vi "Двоич-дес шф.vi"(0 "Registr":T3, 1 "Sign":bool) -> (2 "Segmen 2":T1, 3 "Segmen 1":T2)   [LabVIEW 2017]
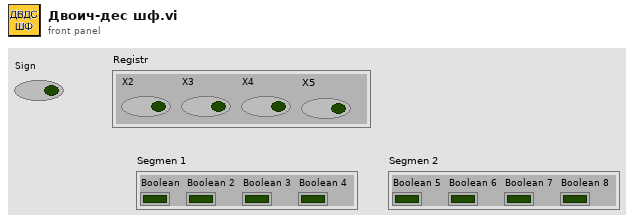
[diagram p1: front panel]
types:
  T1 = cluster{"Boolean 5":bool, "Boolean 6":bool, "Boolean 7":bool, "Boolean 8":bool}
  T2 = cluster{"Boolean":bool, "Boolean 2":bool, "Boolean 3":bool, "Boolean 4":bool}
  T3 = cluster{"X2":bool, "X3":bool, "X4":bool, "X5":bool}
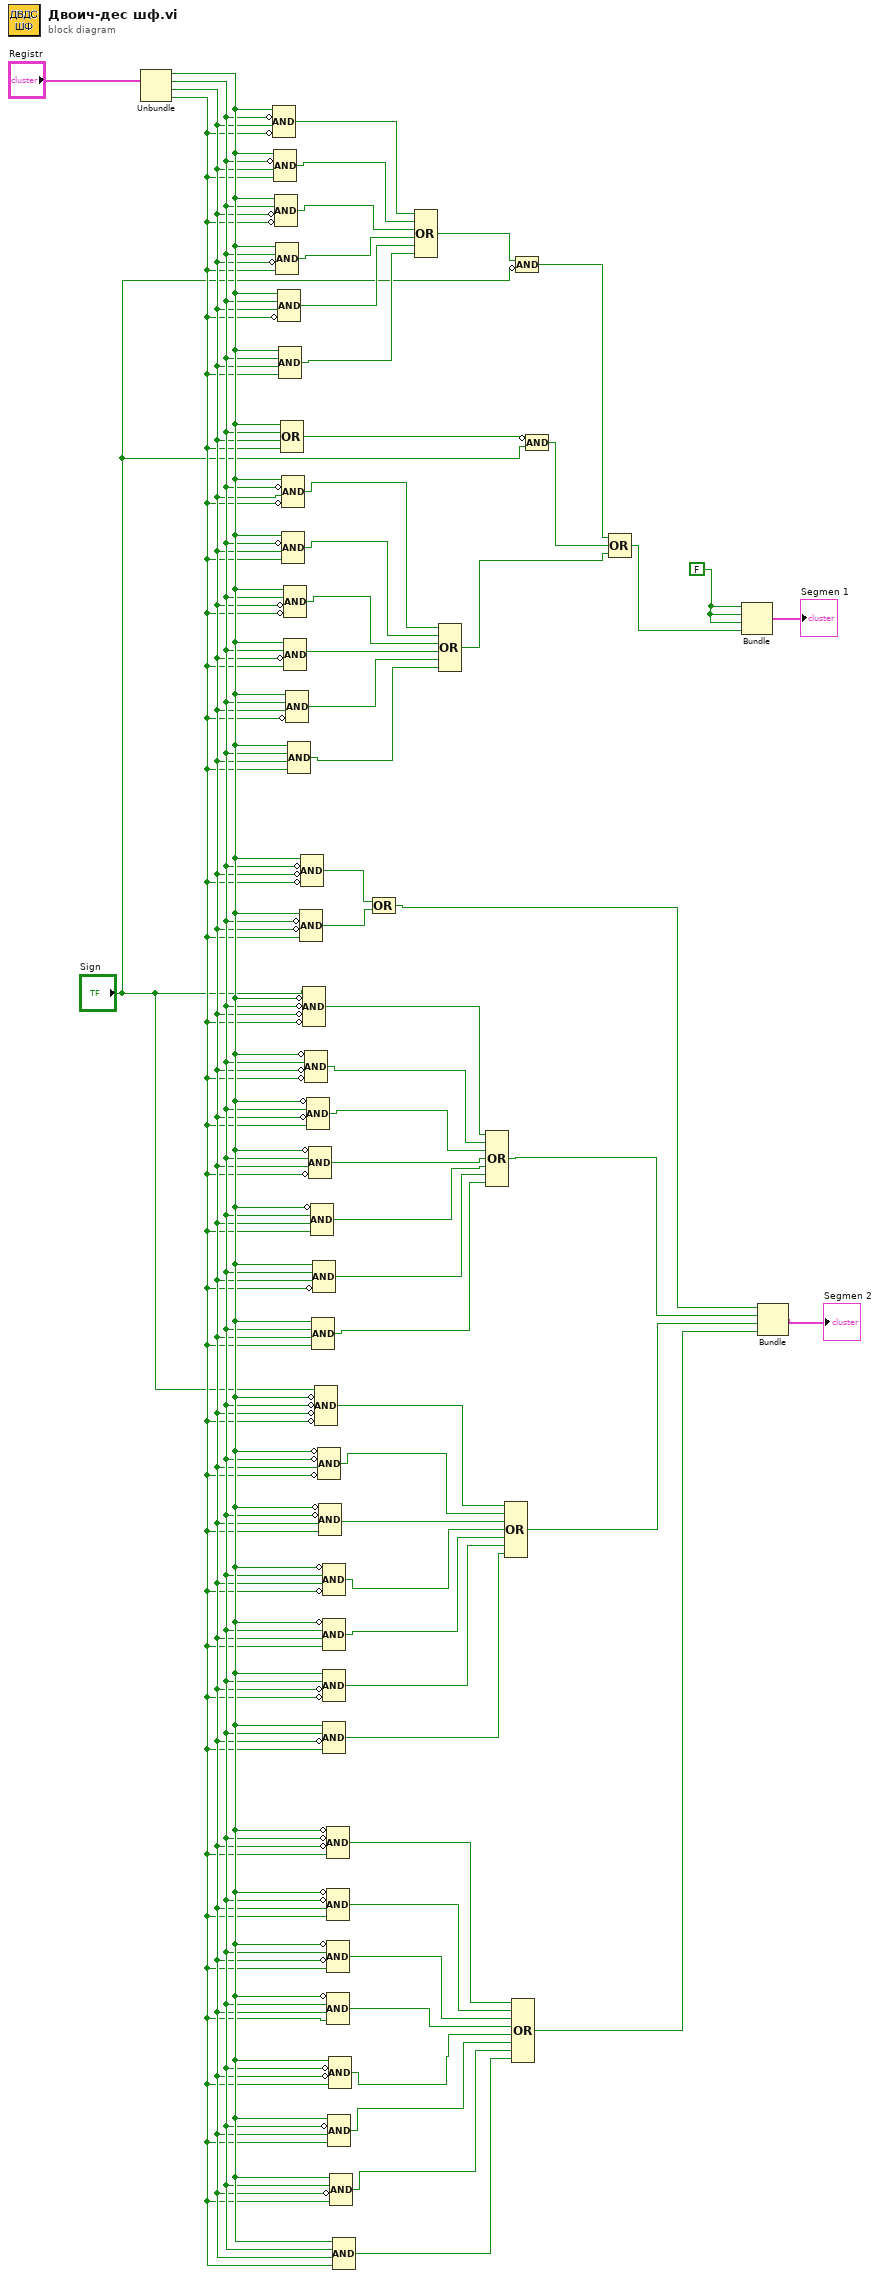
[diagram p0: block diagram]
diagram:
  w11 = FALSE
  n1 = Unbundle("Registr") -> ("X2"=w27:bool, "X3"=w26:bool, "X4"=w25:bool, "X5"=w24:bool)
  n2 = Compound Arithmetic op=AND(w27, invert w26, w25, invert w24) -> (w51:bool)
  n3 = Compound Arithmetic op=AND(w27, invert w26, w25, w24) -> (w50:bool)
  n4 = Compound Arithmetic op=AND(w27, w26, invert w25, invert w24) -> (w49:bool)
  n5 = Compound Arithmetic op=AND(w27, w26, invert w25, w24) -> (w48:bool)
  n6 = Compound Arithmetic op=AND(w27, w26, w25, invert w24) -> (w47:bool)
  n7 = Compound Arithmetic op=AND(w27, w26, w25, w24) -> (w46:bool)
  n8 = Compound Arithmetic op=OR(w27, w26, w25, w24) -> (w13:bool)
  n9 = Compound Arithmetic op=AND(w27, invert w26, w25, invert w24) -> (w6:bool)
  n10 = Compound Arithmetic op=AND(w27, invert w26, w25, w24) -> (w5:bool)
  n11 = Compound Arithmetic op=AND(w27, w26, invert w25, invert w24) -> (w4:bool)
  n12 = Compound Arithmetic op=AND(w27, w26, invert w25, w24) -> (w3:bool)
  n13 = Compound Arithmetic op=AND(w27, w26, w25, invert w24) -> (w2:bool)
  n14 = Compound Arithmetic op=AND(w27, w26, w25, w24) -> (w1:bool)
  n15 = Compound Arithmetic op=AND(w27, invert w26, invert w25, w24) -> (w54:bool)
  n16 = Compound Arithmetic op=AND(w27, invert w26, invert w25, invert w24) -> (w55:bool)
  n17 = Compound Arithmetic op=AND("Sign", invert w27, invert w26, invert w25, invert w24) -> (w42:bool)
  n18 = Compound Arithmetic op=AND(invert w27, w26, invert w25, invert w24) -> (w41:bool)
  n19 = Compound Arithmetic op=AND(invert w27, w26, invert w25, w24) -> (w40:bool)
  n20 = Compound Arithmetic op=AND(invert w27, w26, w25, invert w24) -> (w39:bool)
  n21 = Compound Arithmetic op=AND(invert w27, w26, w25, w24) -> (w38:bool)
  n22 = Compound Arithmetic op=AND(w27, w26, w25, w24) -> (w36:bool)
  n23 = Compound Arithmetic op=AND(w27, w26, w25, invert w24) -> (w37:bool)
  n24 = Compound Arithmetic op=AND("Sign", invert w27, invert w26, invert w25, invert w24) -> (w34:bool)
  n25 = Compound Arithmetic op=AND(invert w27, invert w26, w25, invert w24) -> (w33:bool)
  n26 = Compound Arithmetic op=AND(invert w27, invert w26, w25, w24) -> (w32:bool)
  n27 = Compound Arithmetic op=AND(invert w27, w26, w25, invert w24) -> (w31:bool)
  n28 = Compound Arithmetic op=AND(invert w27, w26, w25, w24) -> (w30:bool)
  n29 = Compound Arithmetic op=AND(w27, w26, invert w25, invert w24) -> (w29:bool)
  n30 = Compound Arithmetic op=AND(w27, w26, invert w25, w24) -> (w28:bool)
  n31 = Compound Arithmetic op=AND(invert w27, invert w26, invert w25, w24) -> (w23:bool)
  n32 = Compound Arithmetic op=AND(invert w27, invert w26, w25, w24) -> (w22:bool)
  n33 = Compound Arithmetic op=AND(invert w27, w26, invert w25, w24) -> (w21:bool)
  n34 = Compound Arithmetic op=AND(invert w27, w26, w25, w24) -> (w20:bool)
  n35 = Compound Arithmetic op=AND(w27, invert w26, w25, w24) -> (w18:bool)
  n36 = Compound Arithmetic op=AND(w27, invert w26, invert w25, w24) -> (w19:bool)
  n37 = Compound Arithmetic op=AND(w27, w26, invert w25, w24) -> (w17:bool)
  n38 = Compound Arithmetic op=AND(w27, w26, w25, w24) -> (w16:bool)
  n39 = Compound Arithmetic op=OR(w55, w54) -> (w44:bool)
  n40 = Compound Arithmetic op=OR(w51, w50, w49, w48, w47, w46) -> (w14:bool)
  n41 = Compound Arithmetic op=OR(w6, w5, w4, w3, w2, w1) -> (w10:bool)
  n42 = Compound Arithmetic op=OR(w42, w41, w40, w39, w38, w37, w36) -> (w43:bool)
  n43 = Compound Arithmetic op=OR(w34, w33, w32, w31, w30, w29, w28) -> (w35:bool)
  n44 = Compound Arithmetic op=OR(w23, w22, w21, w20, w19, w18, w17, w16) -> (w15:bool)
  n45 = Compound Arithmetic op=AND(w14, invert "Sign") -> (w9:bool)
  n46 = Compound Arithmetic op=AND(invert w13, "Sign") -> (w8:bool)
  n47 = Compound Arithmetic op=OR(w9, w8, w10) -> (w7:bool)
  n48 = Bundle(w11, w11, w11, w7) -> (→"Segmen 1":cluster{bool, bool, bool, bool})  [unwired: 1 in]
  n49 = Bundle(w44, w43, w35, w15) -> (→"Segmen 2":cluster{bool, bool, bool, bool})  [unwired: 1 in]
